vi "Begin.vi"() -> (1 "CameraDevRef":T1)   [LabVIEW 2011]
doc: "Called before other user functions, this VI is expected to open initial I/O refnums, load in file data, and do all program initialization. Notice that the <B>error out</B> terminal is simply used for data flow. Wiring it to other structures or subVIs ensures that this VI runs first."
uses:
  <vilib>/Rock Robotics/WPI/Camera/WPI_CameraDevRef.ctl
  <vilib>/Rock Robotics/SystemInterfaces/AI/FPGA_AIChannel.ctl
  <vilib>/Rock Robotics/SystemInterfaces/DIO/FPGA_DIOPWMChannel.ctl
  Robot Global Data.vi
  <vilib>/Rock Robotics/WPI/MotorControl/WPI_MotorControlOpen Jaguar.vi
  <vilib>/Rock Robotics/WPI/MotorControl/WPI_MotorControlOpen Victor.vi
  <vilib>/Rock Robotics/WPI/Joystick/WPI_JoystickDeviceEnum.ctl
  <vilib>/Rock Robotics/SystemInterfaces/DIO/FPGA_DIORelayChannel.ctl
  <vilib>/Rock Robotics/WPI/Relay/WPI_RelayDirection.ctl
  <vilib>/Rock Robotics/SystemInterfaces/Typedef/FPGA_TypedefDigitalModule.ctl
  <vilib>/Rock Robotics/WPI/Counter/WPI_CounterDigitalInputToDigitalSource.vi
  <vilib>/Rock Robotics/SystemInterfaces/DIO/FPGA_DIOChannel.ctl
  <vilib>/Rock Robotics/WPI/Encoder/WPI_EncoderType.ctl
  <vilib>/Rock Robotics/SystemInterfaces/AI/FPGA_AIGyroChannel.ctl
  <vilib>/Rock Robotics/SystemInterfaces/Typedef/FPGA_TypedefAnalogModule.ctl
  <vilib>/Utility/file.llb/Read From Spreadsheet File (DBL).vi
  <vilib>/Rock Robotics/WPI/Relay/WPI_RelayValue.ctl
panel:
  out "AutonArray":dbl[][](array[numeric])
  out "Path and file":string
  in  "Balls In Robot At Start":dbl
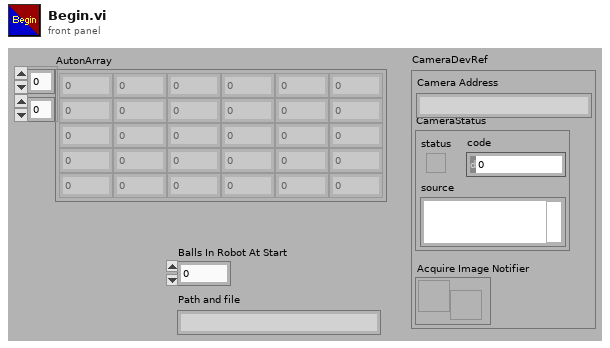
[diagram p1: front panel]
types:
  T1 = typedef "WPI_CameraDevRef.ctl" = cluster{"Camera Address":string, "CameraStatus":errorcluster, "Acquire Image Notifier":refnum<notifier>}
  T2 = typedef "FPGA_DIOPWMChannel.ctl" = enum8{"PWM 1", "PWM 2", "PWM 3", "PWM 4", "PWM 5", "PWM 6", "PWM 7", "PWM 8", "PWM 9", "PWM 10", "Invalid"}
  T3 = typedef "FPGA_AIChannel.ctl" = enum8{"AI 1", "AI 2", "AI 3", "AI 4", "AI 5", "AI 6", "AI 7", "AI 8", "Invalid"}
  T4 = typedef "WPI_CameraImageSize.ctl" = enum16{"640x480", "320x240", "160x120"}
  T5 = cluster{"fps":i32, "compression":i32, "Image Size":T4}
  T6 = typedef "WPI_CameraWhite Balance Values.ctl" = enum16{"Auto", "Fixed indoor", "Fixed outdoor 1", "Fixed outdoor 2", "Fixed fluorescent 1", "Fixed fluorescent 2", "Hold current"}
  T7 = typedef "WPI_CameraExposure Values.ctl" = enum16{"Auto", "Flicker-free 50 Hz", "Flicker-free 60 Hz", "Hold current"}
  T8 = typedef "FPGA_TypedefDigitalModule.ctl" = enum16{"Digital Module 1", "Digital Module 2"}
  T9 = typedef "WPI_ServoDeviceRef.ctl" = cluster{"DeviceStatus":errorcluster, "Digital Module":T8, "PWM Channel":T2, "DeadBand":T10}
  T10 = typedef "WPI_PWMDeadband.ctl" = cluster{"Name":string, "maxPositivePwm":i32, "minPositivePwm":i32, "centerPwm":i32, "maxNegativePwm":i32, "minNegativePwm":i32, "angularRange":u16}
  T11 = typedef "WPI_MotorControlDeviceRef.ctl" = cluster{"DeviceStatus":errorcluster, "Type":enum16{"PWM", "CAN"}, "PWM":cluster{"Digital Module":T8, "PWM Channel":T2, "DeadBand":T10}, "CAN":cluster{"Device Number":u8, "Control Mode":T12, "Semaphore":T13, "Max Vout":dbl}, "Invert":bool, "TransformRef":T14, "InvTransformRef":T14}
  T12 = typedef "WPI_CANJaguar_ControlMode.ctl" = enum8{"Percent VBus", "Current", "Speed", "Position", "Voltage"}
  T13 = typedef "Semaphore RefNum" = refnum<k1>
  T14 = typedef "WPI_PWMTransform_ConPane.ctl" = refnum<vi>
  T15 = typedef "WPI_RelayValue.ctl" = enum16{"Off", "On", "Forward", "Reverse"}
  T16 = typedef "FPGA_DIORelayChannel.ctl" = enum8{"Relay 1", "Relay 2", "Relay 3", "Relay 4", "Relay 5", "Relay 6", "Relay 7", "Relay 8", "Invalid"}
  T17 = typedef "WPI_RelayDirection.ctl" = enum16{"Both directions", "Forward only", "Reverse only"}
  T18 = typedef "WPI_JoystickDeviceEnum.ctl" = enum16{"USB 1", "USB 2", "USB 3", "USB 4", "Kinect 1", "Kinect 2"}
  T19 = typedef "WPI_JoystickDevRef.ctl" = cluster{"Device":T18}
  T20 = typedef "WPI_RelayDevRef.ctl" = cluster{"DevStatus":errorcluster, "Relay Channel":T16, "Digital Module":T8, "Relay Direction":T17}
  T21 = typedef "WPI_AnalogChannelDevRef.ctl" = cluster{"DevStatus":errorcluster, "Analog Module":T22, "Analog Channel":T3}
  T22 = typedef "FPGA_TypedefAnalogModule.ctl" = enum16{"Analog Module 1", "Analog Module 2"}
  T23 = typedef "FPGA_AIGyroChannel.ctl" = enum8{"AI 1", "AI 2", "Invalid"}
  T24 = typedef "WPI_EncoderType.ctl" = enum16{"1x", "2x", "4x"}
  T25 = typedef "FPGA_DIOChannel.ctl" = enum8{"DIO 1", "DIO 2", "DIO 3", "DIO 4", "DIO 5", "DIO 6", "DIO 7", "DIO 8", "DIO 9", "DIO 10", "DIO 11", "DIO 12", "DIO 13", "DIO 14", "Invalid"}
  T26 = typedef "WPI_DigitalInputDevRef.ctl" = cluster{"DevStatus":errorcluster, "DIO Channel":T25, "Digital Module":T8}
  T27 = typedef "FPGA_CounterEncoderSourceConvertionLVSourceType.ctl" = cluster{"DevStatus":errorcluster, "AnalogTriggerMode?":bool, "DigitalMode":cluster{"Digital Module":T8, "DIO Channel":T28}, "AnalogTriggerMode":cluster{"AnalogTriggerIndex":T29, "OutputType":T30}}
  T28 = typedef "FPGA_DIODigitalSourceChannel.ctl" = enum8{"DIO 1", "DIO 2", "DIO 3", "DIO 4", "DIO 5", "DIO 6", "DIO 7", "DIO 8", "DIO 9", "DIO 10", "DIO 11", "DIO 12", "DIO 13", "DIO 14", "Disabled"}
  T29 = typedef "FPGA_AnalogTriggerIndex.ctl" = enum8{"Trig 0", "Trig 1", "Trig 2", "Trig 3", "Trig 4", "Trig 5", "Trig 6", "Trig 7", "Invalid"}
  T30 = typedef "FPGA_AnalogTriggerOutType.ctl" = enum16{"InWindow", "TriggerState", "Rising", "Falling"}
  T31 = typedef "WPI_EncoderDevRef.ctl" = cluster{"DevStatus":errorcluster, "EncoderIndex":T32, "CounterIndex":T33, "DistancePerCount":dbl, "Decoding Type":T24}
  T32 = typedef "FPGA_EncoderIdx.ctl" = enum8{"Enc 0", "Enc 1", "Enc 2", "Enc 3", "Invalid"}
  T33 = typedef "FPGA_CounterCtrSystemIndex.ctl" = enum8{"Ctr 0", "Ctr 1", "Ctr 2", "Ctr 3", "Ctr 4", "Ctr 5", "Ctr 6", "Ctr 7", "Invalid"}
  T34 = typedef "WPI_GyroDevRef.ctl" = cluster{"DevStatus":errorcluster, "Analog Module":T22, "Analog Channel":T3, "Offset":dbl, "Gain (VoltsPerDegree/Second)":dbl}
  T35 = typedef "WPI_UltrasonicDeviceRef.ctl" = cluster{"DevStatus":errorcluster, "Ping Digital Module":T8, "Echo Digital Module":T8, "Ping Channel":T25, "Echo Channel":T25, "CntIndex":T33}
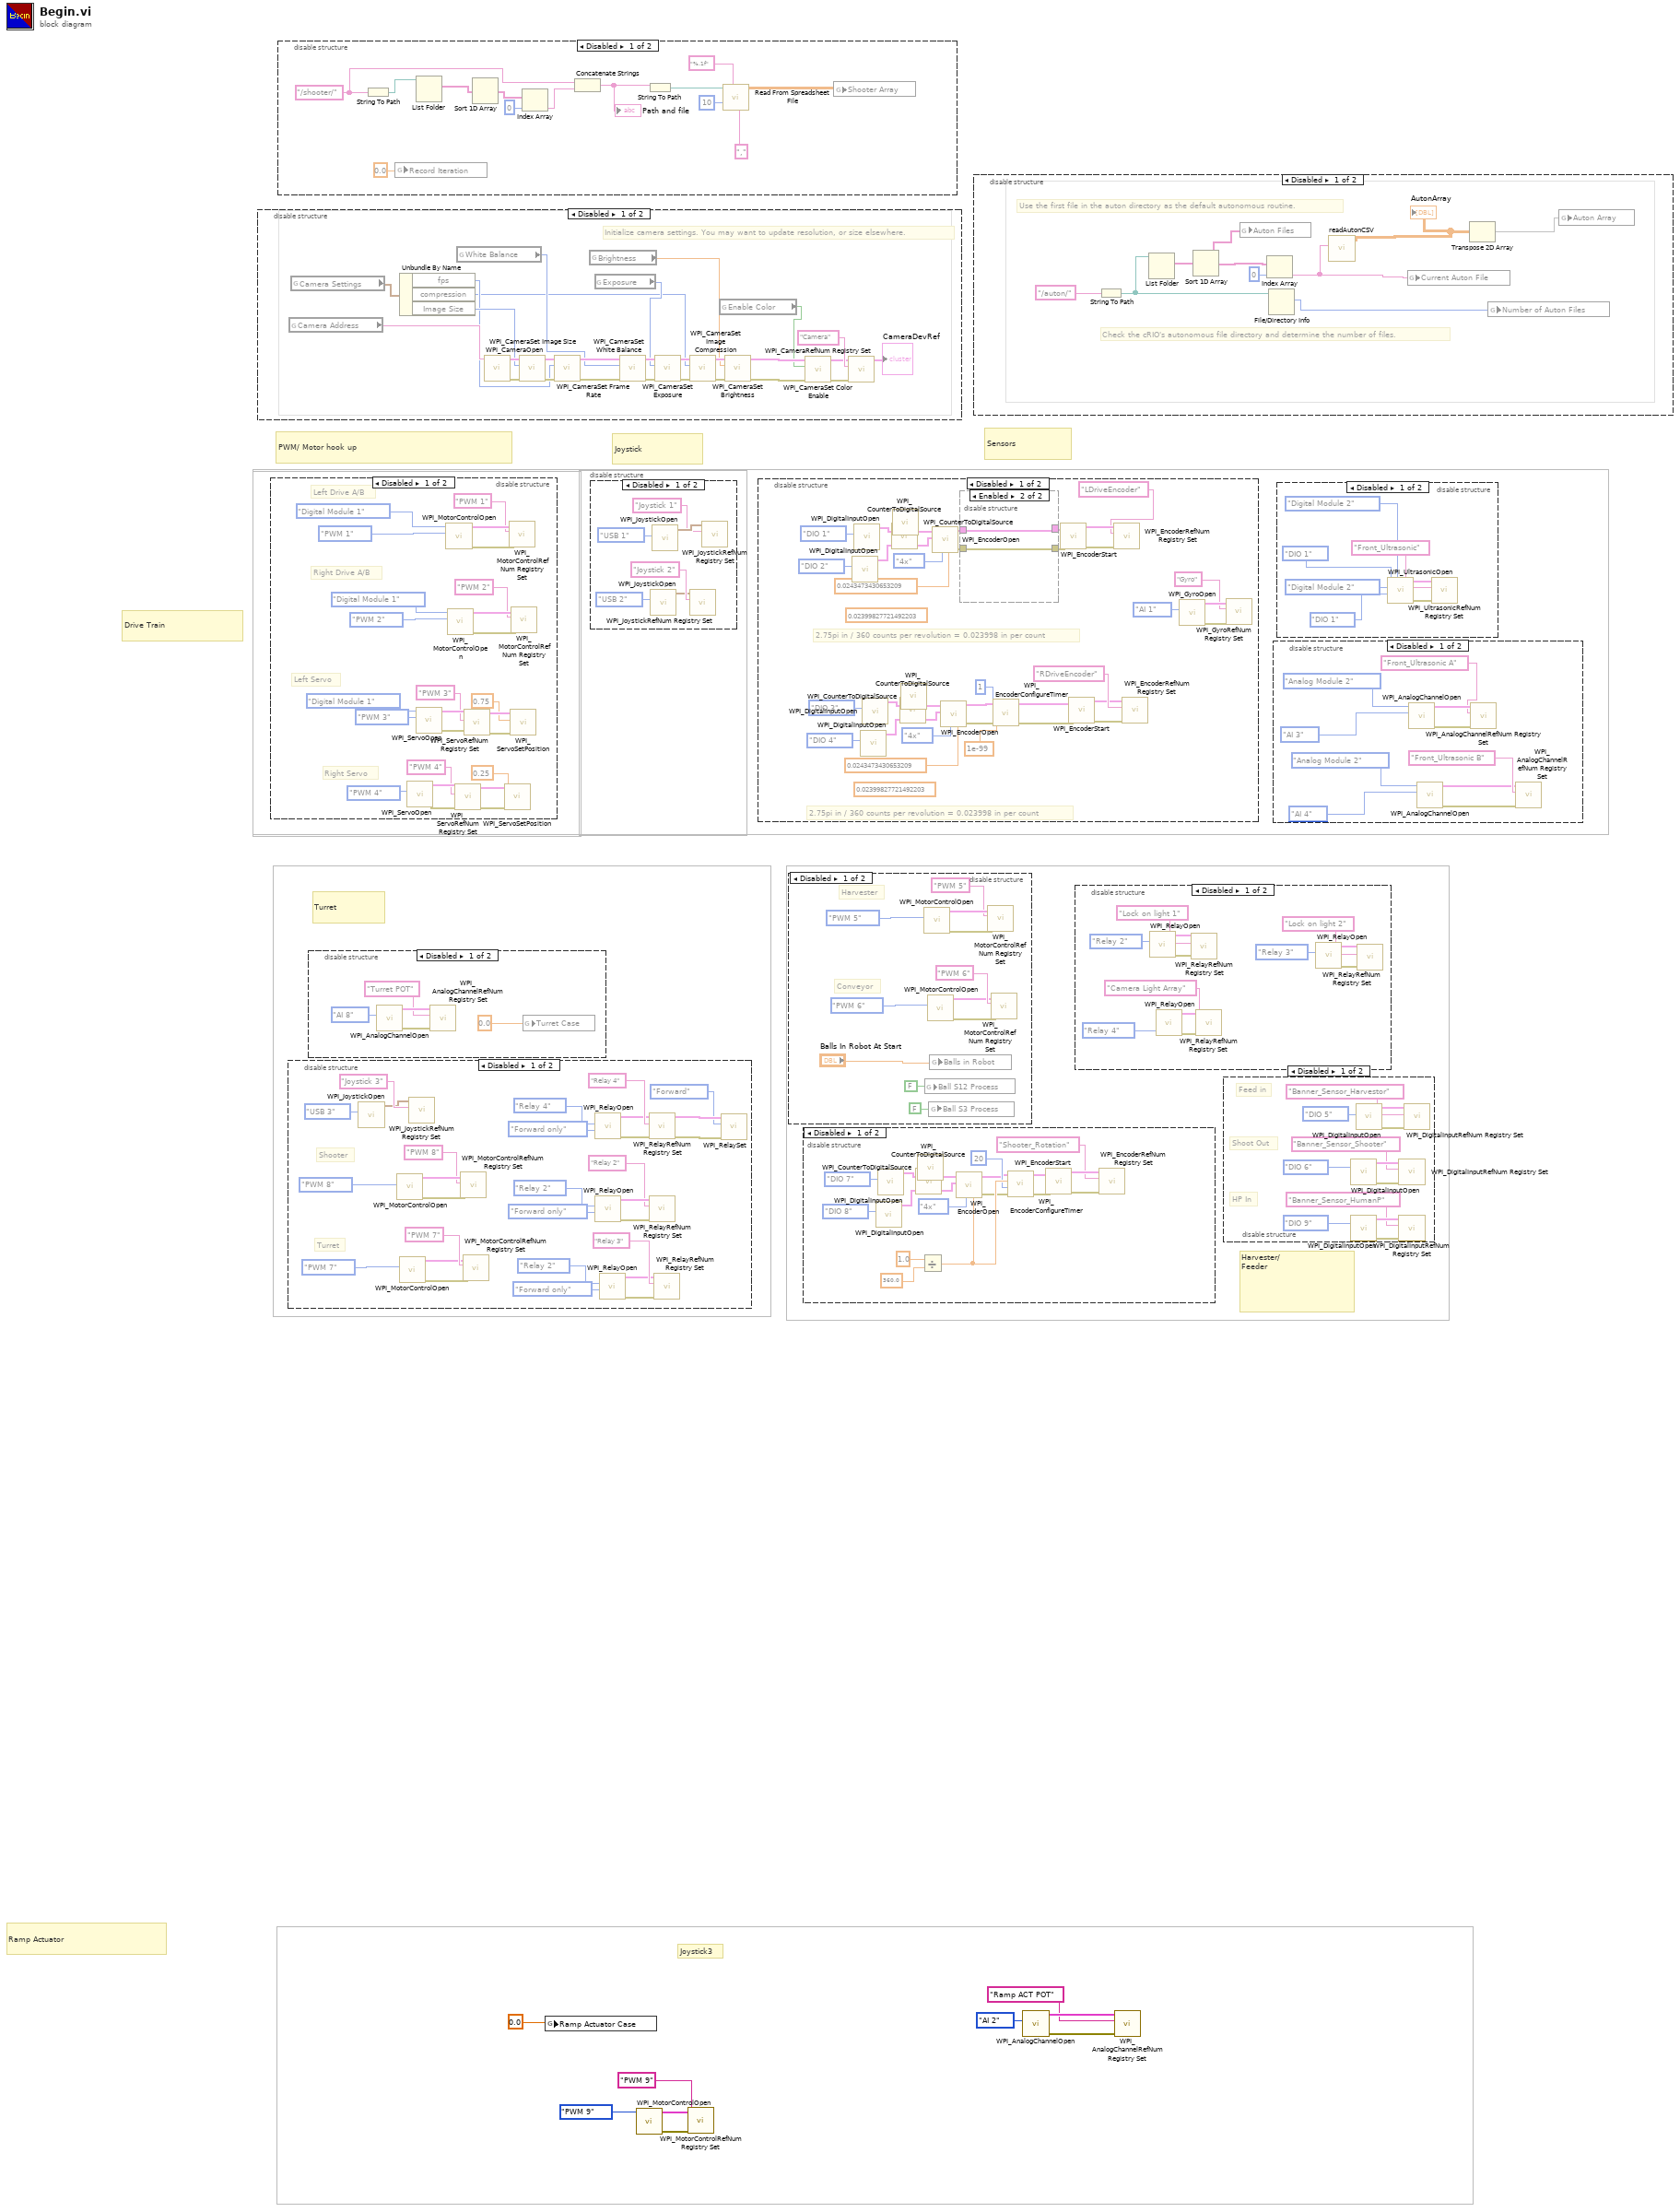
[diagram p0: block diagram]
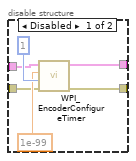
[diagram p9: hidden frame]
diagram:
  # "Harvester/\nFeeder"
  # "Joystick3"
  # "Turret"
  # "Ramp Actuator"
  # "Drive Train"
  # "Sensors"
  # "Joystick"
  # "PWM/ Motor hook up"
  n1 = disable-structure shown="Disabled" {
    frame Disabled {
      # "Initialize camera settings. You may want to update resolution, or size elsewhere."
      n2 = global read "Robot Global Data.vi" "Camera Address"() -> (w23:string)
      n3 = global read "Robot Global Data.vi" "Camera Settings"() -> (w22:T5)
      n4 = Unbundle By Name(w22) -> ("fps"=w20:i32, "compression"=w17:i32, "Image Size"=w21:T4)
      n5 = global read "Robot Global Data.vi" "White Balance"() -> (w19:T6)
      n6 = call <vilib>:"WPI_CameraOpen.vi"("Camera Address"=w23) -> ("error out"=w29:errorcluster, "CameraDevRef"=w30:T1)  [unwired: 1 in, 8 out]
      n7 = call <vilib>:"WPI_CameraSet Image Size.vi"("error in (no error)"=w29, "Image Size"=w21, "CameraDevRef"=w30) -> ("error out"=w28:errorcluster, "CameraDevRef Out"=w31:T1)  [unwired: 7 out]
      n8 = call <vilib>:"WPI_CameraSet Frame Rate.vi"("error in (no error)"=w28, "Frame Rate (fps)"=w20, "CameraDevRef"=w31) -> ("error out"=w27:errorcluster, "CameraDevRef Out"=w33:T1)  [unwired: 7 out]
      n9 = global read "Robot Global Data.vi" "Brightness"() -> (w16:dbl)
      n10 = global read "Robot Global Data.vi" "Exposure"() -> (w18:T7)
      n11 = call <vilib>:"WPI_CameraSet White Balance.vi"("error in (no error)"=w27, "White Balance"=w19, "CameraDevRef"=w33) -> ("error out"=w26:errorcluster, "CameraDevRef Out"=w32:T1)  [unwired: 7 out]
      n12 = call <vilib>:"WPI_CameraSet Exposure.vi"("error in (no error)"=w26, "Exposure"=w18, "CameraDevRef"=w32) -> ("error out"=w25:errorcluster, "CameraDevRef Out"=w35:T1)  [unwired: 7 out]
      n13 = call <vilib>:"WPI_CameraSet Image Compression.vi"("error in (no error)"=w25, "Compression"=w17, "CameraDevRef"=w35) -> ("error out"=w24:errorcluster, "CameraDevRef Out"=w34:T1)  [unwired: 7 out]
      n14 = global read "Robot Global Data.vi" "Enable Color"() -> (w11:bool)
      n15 = call <vilib>:"WPI_CameraSet Brightness.vi"("error in (no error)"=w24, "Brightness"=w16, "CameraDevRef"=w34) -> ("error out"=w14:errorcluster, "CameraDevRef Out"=w15:T1)  [unwired: 7 out]
      n16 = call <vilib>:"WPI_CameraSet Color Enable.vi"("error in (no error)"=w14, "Color Enabled"=w11, "CameraDevRef"=w15) -> ("error out"=w12:errorcluster, "CameraDevRef Out"=w13:T1)  [unwired: 7 in]
      n17 = call <vilib>:"WPI_CameraRefNum Registry Set.vi"("error in (no error)"=w12, "refnum name"="Camera", "CameraDevRef"=w13) -> ("CameraDevRef"=→"CameraDevRef":T1)  [unwired: 8 out]
    }
    frame Enabled {
    }
  }
  n18 = disable-structure shown="Disabled" {
    frame Disabled {
      # "Right Drive A/B"
      # "Left Drive A/B"
      # "Right Servo"
      # "Left Servo"
      n19 = call <vilib>:"WPI_ServoOpen.vi"("PWM Channel"=FPGA_DIOPWMChannel."PWM 4") -> ("error out"=w43:errorcluster, "ServoDeviceRef"=w58:T9)  [unwired: 9 in]
      n20 = call <vilib>:"WPI_ServoOpen.vi"("PWM Channel"=FPGA_DIOPWMChannel."PWM 3", "Digital Module (Module 1)"=FPGA_TypedefDigitalModule."Digital Module 1") -> ("error out"=w44:errorcluster, "ServoDeviceRef"=w60:T9)  [unwired: 8 in]
      n21 = call-poly <vilib>:"WPI_MotorControlOpen.vi"("PWM Channel"=FPGA_DIOPWMChannel."PWM 1", "Digital Module (Module 1)"=FPGA_TypedefDigitalModule."Digital Module 1") -> ("error out"=w48:errorcluster, "MotorControlDeviceRef"=w51:T11)  [unwired: 8 in]
      n22 = call-poly <vilib>:"WPI_MotorControlOpen.vi"("PWM Channel"=FPGA_DIOPWMChannel."PWM 2", "Digital Module (Module 1)"=FPGA_TypedefDigitalModule."Digital Module 1") -> ("error out"=w49:errorcluster, "MotorControlDeviceRef"=w54:T11)  [unwired: 8 in]
      n23 = call <vilib>:"WPI_ServoRefNum Registry Set.vi"("error in (no error)"=w43, "refnum name"="PWM 4", "ServoDeviceRef"=w58) -> ("error out"=w41:errorcluster, "ServoDeviceRef"=w42:T9)  [unwired: 7 in]
      n24 = call <vilib>:"WPI_ServoRefNum Registry Set.vi"("error in (no error)"=w44, "refnum name"="PWM 3", "ServoDeviceRef"=w60) -> ("error out"=w39:errorcluster, "ServoDeviceRef"=w40:T9)  [unwired: 7 in]
      n25 = call <vilib>:"WPI_ServoSetPosition.vi"("error in (no error)"=w41, "Position"=0.25, "ServoDeviceRef"=w42) -> ()  [unwired: 7 in, 2 out]
      n26 = call <vilib>:"WPI_MotorControlRefNum Registry Set.vi"("error in (no error)"=w48, "refnum name"="PWM 1", "MotorControlDevRef"=w51) -> ()  [unwired: 7 in, 2 out]
      n27 = call <vilib>:"WPI_ServoSetPosition.vi"("error in (no error)"=w39, "Position"=0.75, "ServoDeviceRef"=w40) -> ()  [unwired: 7 in, 2 out]
      n28 = call <vilib>:"WPI_MotorControlRefNum Registry Set.vi"("error in (no error)"=w49, "refnum name"="PWM 2", "MotorControlDevRef"=w54) -> ()  [unwired: 7 in, 2 out]
    }
    frame Enabled {
    }
  }
  n29 = disable-structure shown="Disabled" {
    frame Disabled {
      w65 = "/shooter/" ("string")
      n30 = String To Path(string=w65) -> (path=w74:path)
      n31 = global write "Robot Global Data.vi" "Record Iteration"(0.0 ("Record Iteration")) -> ()
      n32 = List Folder(path=w74) -> (filenames=w73:string[])  [unwired: 1 in, 5 out]
      n33 = Sort 1D Array(array=w73) -> (sorted array=w72:string[])
      n34 = Index Array(array=w72, index=0) -> (element=w64:string)
      n35 = Concatenate Strings(w65, w64) -> (w67:string)
      "Path and file" <- w67
      n36 = String To Path(string=w67) -> (path=w66:path)
      n37 = call-poly <vilib>:"Read From Spreadsheet File.vi"("delimiter (\\t)"="," ("delimiter (\\t)"), "format (%.3f)"="%.1f", "number of rows (all:-1)"=10, "file path (dialog if empty)"=w66) -> ("all rows"=w63:dbl[][])  [unwired: 1 in, 6 out]
      n38 = global write "Robot Global Data.vi" "Shooter Array"(w63) -> ()
    }
    frame Enabled {
    }
  }
  n39 = disable-structure shown="Disabled" {
    frame Disabled {
      # "Turret"
      # "Shooter"
      n40 = call <vilib>:"WPI_JoystickOpen.vi"("JoystickDevice"=WPI_JoystickDeviceEnum."USB 3") -> ("JoystickDevRef"=w102:T19)  [unwired: 10 in]
      n41 = call-poly <vilib>:"WPI_MotorControlOpen.vi"("PWM Channel"=FPGA_DIOPWMChannel."PWM 8") -> ("error out"=w79:errorcluster, "MotorControlDeviceRef"=w81:T11)  [unwired: 9 in]
      n42 = call-poly <vilib>:"WPI_MotorControlOpen.vi"("PWM Channel"=FPGA_DIOPWMChannel."PWM 7") -> ("error out"=w78:errorcluster, "MotorControlDeviceRef"=w76:T11)  [unwired: 9 in]
      n43 = call <vilib>:"WPI_JoystickRefNum Registry Set.vi"("refnum name"="Joystick 3", "JoystickDevRef"=w102) -> ()  [unwired: 8 in, 2 out]
      n44 = call <vilib>:"WPI_MotorControlRefNum Registry Set.vi"("error in (no error)"=w79, "refnum name"="PWM 8", "MotorControlDevRef"=w81) -> ()  [unwired: 7 in, 2 out]
      n45 = call <vilib>:"WPI_MotorControlRefNum Registry Set.vi"("error in (no error)"=w78, "refnum name"="PWM 7", "MotorControlDevRef"=w76) -> ()  [unwired: 7 in, 2 out]
      n46 = call <vilib>:"WPI_RelayOpen.vi"("Relay Direction"=WPI_RelayDirection."Forward only", "Relay Channel"=FPGA_DIORelayChannel."Relay 4") -> ("error out"=w87:errorcluster, "RelayDevRef"=w86:T20)  [unwired: 8 in]
      n47 = call <vilib>:"WPI_RelayOpen.vi"("Relay Direction"=WPI_RelayDirection."Forward only", "Relay Channel"=FPGA_DIORelayChannel."Relay 2") -> ("error out"=w99:errorcluster, "RelayDevRef"=w100:T20)  [unwired: 8 in]
      n48 = call <vilib>:"WPI_RelayOpen.vi"("Relay Direction"=WPI_RelayDirection."Forward only", "Relay Channel"=FPGA_DIORelayChannel."Relay 2") -> ("error out"=w92:errorcluster, "RelayDevRef"=w91:T20)  [unwired: 8 in]
      n49 = call <vilib>:"WPI_RelayRefNum Registry Set.vi"("error in (no error)"=w87, "refnum name"="Relay 4", "RelayDevRef"=w86) -> ("error out"=w84:errorcluster, "RelayDevRef"=w85:T20)  [unwired: 7 in]
      n50 = call <vilib>:"WPI_RelayRefNum Registry Set.vi"("error in (no error)"=w99, "refnum name"="Relay 2", "RelayDevRef"=w100) -> ()  [unwired: 7 in, 2 out]
      n51 = call <vilib>:"WPI_RelayRefNum Registry Set.vi"("error in (no error)"=w92, "refnum name"="Relay 3", "RelayDevRef"=w91) -> ()  [unwired: 7 in, 2 out]
      n52 = call <vilib>:"WPI_RelaySet.vi"("error in (no error)"=w84, "RelayValue"=WPI_RelayValue."Forward", "RelayDevRef"=w85) -> ()  [unwired: 7 in, 2 out]
    }
    frame Enabled {
    }
  }
  n53 = disable-structure shown="Disabled" {
    frame Disabled {
      n54 = call <vilib>:"WPI_AnalogChannelOpen.vi"("Analog Channel"=FPGA_AIChannel."AI 8") -> ("error out"=w107:errorcluster, "AIDeviceRef"=w108:T21)  [unwired: 9 in]
      n55 = call <vilib>:"WPI_AnalogChannelRefNum Registry Set.vi"("error in (no error)"=w107, "refnum name"="Turret POT", "AIDeviceRef"=w108) -> ()  [unwired: 7 in, 2 out]
      n56 = global write "Robot Global Data.vi" "Turret Case"(0.0 ("Return To Home Case")) -> ()
    }
    frame Enabled {
    }
  }
  n57 = global write "Robot Global Data.vi" "Ramp Actuator Case"(0.0 ("Ramp Actuator Case")) -> ()
  n58 = disable-structure shown="Disabled" {
    frame Disabled {
      n59 = call <vilib>:"WPI_JoystickOpen.vi"("JoystickDevice"=WPI_JoystickDeviceEnum."USB 2") -> ("JoystickDevRef"=w111:T19)  [unwired: 10 in]
      n60 = call <vilib>:"WPI_JoystickOpen.vi"("JoystickDevice"=WPI_JoystickDeviceEnum."USB 1") -> ("JoystickDevRef"=w114:T19)  [unwired: 10 in]
      n61 = call <vilib>:"WPI_JoystickRefNum Registry Set.vi"("refnum name"="Joystick 2", "JoystickDevRef"=w111) -> ()  [unwired: 8 in, 2 out]
      n62 = call <vilib>:"WPI_JoystickRefNum Registry Set.vi"("refnum name"="Joystick 1", "JoystickDevRef"=w114) -> ()  [unwired: 8 in, 2 out]
    }
    frame Enabled {
    }
  }
  n63 = call-poly <vilib>:"WPI_MotorControlOpen.vi"("PWM Channel"=FPGA_DIOPWMChannel."PWM 9") -> ("error out"=w3:errorcluster, "MotorControlDeviceRef"=w4:T11)  [unwired: 9 in]
  n64 = call <vilib>:"WPI_MotorControlRefNum Registry Set.vi"("error in (no error)"=w3, "refnum name"="PWM 9", "MotorControlDevRef"=w4) -> ()  [unwired: 7 in, 2 out]
  n65 = disable-structure shown="Disabled" {
    frame Disabled {
      (unwired) 0.02399827721492203 ("DistancePerCount")
      (unwired) 0.02399827721492203 ("DistancePerCount")
      # "2.75pi in / 360 counts per revolution = 0.023998 in per count"
      # "2.75pi in / 360 counts per revolution = 0.023998 in per count"
      n66 = call <vilib>:"WPI_DigitalInputOpen.vi"("DIO Channel"=FPGA_DIOChannel."DIO 2") -> ("DigitalInputDevRef"=w142:T26)  [unwired: 9 in, 1 out]
      n67 = call <vilib>:"WPI_DigitalInputOpen.vi"("DIO Channel"=FPGA_DIOChannel."DIO 1") -> ("DigitalInputDevRef"=w139:T26)  [unwired: 9 in, 1 out]
      n68 = call <vilib>:"WPI_DigitalInputOpen.vi"("DIO Channel"=FPGA_DIOChannel."DIO 4") -> ("DigitalInputDevRef"=w133:T26)  [unwired: 9 in, 1 out]
      n69 = call <vilib>:"WPI_DigitalInputOpen.vi"("DIO Channel"=FPGA_DIOChannel."DIO 3") -> ("DigitalInputDevRef"=w136:T26)  [unwired: 9 in, 1 out]
      n70 = call-poly <vilib>:"WPI_CounterToDigitalSource.vi"("DigitalInputDevRef"=w142) -> ("Digital Source"=w143:T27)  [unwired: 6 in]
      n71 = call-poly <vilib>:"WPI_CounterToDigitalSource.vi"("DigitalInputDevRef"=w139) -> ("Digital Source"=w138:T27)  [unwired: 6 in]
      n72 = call-poly <vilib>:"WPI_CounterToDigitalSource.vi"("DigitalInputDevRef"=w133) -> ("Digital Source"=w132:T27)  [unwired: 6 in]
      n73 = call-poly <vilib>:"WPI_CounterToDigitalSource.vi"("DigitalInputDevRef"=w136) -> ("Digital Source"=w137:T27)  [unwired: 6 in]
      n74 = call <vilib>:"WPI_EncoderOpen.vi"("DistancePerCount"=0.0243473430653209, "Decoding Type"=WPI_EncoderType."4x", "BSource"=w143, "ASource"=w138) -> ("error out"=w145:errorcluster, "EncoderDevRef"=w146:T31)  [unwired: 6 in]
      n75 = call <vilib>:"WPI_EncoderOpen.vi"("DistancePerCount"=0.0243473430653209, "Decoding Type"=WPI_EncoderType."4x", "BSource"=w132, "ASource"=w137) -> ("error out"=w129:errorcluster, "EncoderDevRef"=w128:T31)  [unwired: 6 in]
      n76 = disable-structure shown="Enabled" {
        disable-tunnel: [w156 w157] -> w148
        disable-tunnel: [w155 w158] -> w147
        disable-tunnel: w146 -> [w152 w158]
        disable-tunnel: w145 -> [w151 w157]
        frame Disabled {
          n77 = call <vilib>:"WPI_EncoderConfigureTimer.vi"("error in (no error)"=w151, "Number Samples to Average"=u8 1, "Minimum Rate"=1e-99, "EncoderDevRef"=w152) -> ("error out"=w156:errorcluster, "EncoderDevRef"=w155:T31)  [unwired: 6 in]
        }
        frame Enabled {
        }
      }
      n78 = call <vilib>:"WPI_EncoderConfigureTimer.vi"("error in (no error)"=w129, "Number Samples to Average"=u8 1, "Minimum Rate"=1e-99, "EncoderDevRef"=w128) -> ("error out"=w124:errorcluster, "EncoderDevRef"=w125:T31)  [unwired: 6 in]
      n79 = call <vilib>:"WPI_EncoderStart.vi"("error in (no error)"=w148, "EncoderDevRef"=w147) -> ("error out"=w150:errorcluster, "EncoderDevRef"=w149:T31)  [unwired: 8 in]
      n80 = call <vilib>:"WPI_EncoderStart.vi"("error in (no error)"=w124, "EncoderDevRef"=w125) -> ("error out"=w122:errorcluster, "EncoderDevRef"=w123:T31)  [unwired: 8 in]
      n81 = call <vilib>:"WPI_EncoderRefNum Registry Set.vi"("error in (no error)"=w150, "refnum name"="LDriveEncoder", "EncoderDevRef"=w149) -> ()  [unwired: 7 in, 2 out]
      n82 = call <vilib>:"WPI_EncoderRefNum Registry Set.vi"("error in (no error)"=w122, "refnum name"="RDriveEncoder", "EncoderDevRef"=w123) -> ()  [unwired: 7 in, 2 out]
      n83 = call <vilib>:"WPI_GyroOpen.vi"("Analog Channel"=FPGA_AIGyroChannel."AI 1") -> ("error out"=w118:errorcluster, "GyroDevRef"=w117:T34)  [unwired: 8 in, 1 out]
      n84 = call <vilib>:"WPI_GyroRefNum Registry Set.vi"("error in (no error)"=w118, "refnum name"="Gyro", "GyroDevRef"=w117) -> ()  [unwired: 7 in, 2 out]
    }
    frame Enabled {
    }
  }
  n85 = disable-structure shown="Disabled" {
    frame Disabled {
      # "Harvester"
      # "Conveyor"
      n86 = call-poly <vilib>:"WPI_MotorControlOpen.vi"("PWM Channel"=FPGA_DIOPWMChannel."PWM 5") -> ("error out"=w166:errorcluster, "MotorControlDeviceRef"=w168:T11)  [unwired: 9 in]
      n87 = global write "Robot Global Data.vi" "Ball S12 Process"(FALSE ("Ball S12 Process")) -> ()
      n88 = call-poly <vilib>:"WPI_MotorControlOpen.vi"("PWM Channel"=FPGA_DIOPWMChannel."PWM 6") -> ("error out"=w165:errorcluster, "MotorControlDeviceRef"=w163:T11)  [unwired: 9 in]
      n89 = global write "Robot Global Data.vi" "Ball S3 Process"(FALSE ("Ball S3 Process")) -> ()
      n90 = global write "Robot Global Data.vi" "Balls in Robot"("Balls In Robot At Start") -> ()
      n91 = call <vilib>:"WPI_MotorControlRefNum Registry Set.vi"("error in (no error)"=w166, "refnum name"="PWM 5", "MotorControlDevRef"=w168) -> ()  [unwired: 7 in, 2 out]
      n92 = call <vilib>:"WPI_MotorControlRefNum Registry Set.vi"("error in (no error)"=w165, "refnum name"="PWM 6", "MotorControlDevRef"=w163) -> ()  [unwired: 7 in, 2 out]
    }
    frame Enabled {
    }
  }
  n93 = disable-structure shown="Disabled" {
    frame Disabled {
      n94 = call <vilib>:"WPI_DigitalInputOpen.vi"("DIO Channel"=FPGA_DIOChannel."DIO 8") -> ("DigitalInputDevRef"=w174:T26)  [unwired: 9 in, 1 out]
      n95 = call <vilib>:"WPI_DigitalInputOpen.vi"("DIO Channel"=FPGA_DIOChannel."DIO 7") -> ("DigitalInputDevRef"=w171:T26)  [unwired: 9 in, 1 out]
      n96 = call-poly <vilib>:"WPI_CounterToDigitalSource.vi"("DigitalInputDevRef"=w174) -> ("Digital Source"=w175:T27)  [unwired: 6 in]
      n97 = call-poly <vilib>:"WPI_CounterToDigitalSource.vi"("DigitalInputDevRef"=w171) -> ("Digital Source"=w170:T27)  [unwired: 6 in]
      n98 = Divide(x=1.0, y=360.0) -> (x/y=w187:dbl)
      n99 = call <vilib>:"WPI_EncoderOpen.vi"("DistancePerCount"=w187, "Decoding Type"=WPI_EncoderType."4x", "BSource"=w175, "ASource"=w170) -> ("error out"=w178:errorcluster, "EncoderDevRef"=w179:T31)  [unwired: 6 in]
      n100 = call <vilib>:"WPI_EncoderConfigureTimer.vi"("error in (no error)"=w178, "Number Samples to Average"=u8 20, "Minimum Rate"=w187, "EncoderDevRef"=w179) -> ("error out"=w182:errorcluster, "EncoderDevRef"=w181:T31)  [unwired: 6 in]
      n101 = call <vilib>:"WPI_EncoderStart.vi"("error in (no error)"=w182, "EncoderDevRef"=w181) -> ("error out"=w184:errorcluster, "EncoderDevRef"=w183:T31)  [unwired: 8 in]
      n102 = call <vilib>:"WPI_EncoderRefNum Registry Set.vi"("error in (no error)"=w184, "refnum name"="Shooter_Rotation", "EncoderDevRef"=w183) -> ()  [unwired: 7 in, 2 out]
    }
    frame Enabled {
    }
  }
  n103 = disable-structure shown="Disabled" {
    frame Disabled {
      # "Check the cRIO's autonomous file directory and determine the number of files."
      # "Use the first file in the auton directory as the default autonomous routine."
      n104 = String To Path(string="/auton/") -> (path=w195:path)
      n105 = List Folder(path=w195) -> (filenames=w194:string[])  [unwired: 1 in, 5 out]
      n106 = Sort 1D Array(array=w194) -> (sorted array=w190:string[])
      n107 = global write "Robot Global Data.vi" "Auton Files"(w190) -> ()
      n108 = Index Array(array=w190, index=0) -> (element=w191:string)
      n109 = File/Directory Info(path=w195) -> (size=w192:i64)  [unwired: 1 in, 6 out]
      n110 = call "readAutonCSV.vi"("AutonFile"=w191) -> ("AutonArray"=w189:dbl[][])  [unwired: 7 in]
      "AutonArray" <- w189
      n111 = global write "Robot Global Data.vi" "Current Auton File"(w191) -> ()
      n112 = Transpose 2D Array(2D array=w189) -> (transposed array=w188:dbl[][])
      n113 = global write "Robot Global Data.vi" "Number of Auton Files"(w192) -> ()
      n114 = global write "Robot Global Data.vi" "Auton Array"(w188) -> ()
    }
    frame Enabled {
    }
  }
  n115 = call <vilib>:"WPI_AnalogChannelOpen.vi"("Analog Channel"=FPGA_AIChannel."AI 2") -> ("error out"=w8:errorcluster, "AIDeviceRef"=w9:T21)  [unwired: 9 in]
  n116 = disable-structure shown="Disabled" {
    frame Disabled {
      n117 = call <vilib>:"WPI_RelayOpen.vi"("Relay Channel"=FPGA_DIORelayChannel."Relay 2") -> ("error out"=w206:errorcluster, "RelayDevRef"=w205:T20)  [unwired: 9 in]
      n118 = call <vilib>:"WPI_RelayOpen.vi"("Relay Channel"=FPGA_DIORelayChannel."Relay 4") -> ("error out"=w208:errorcluster, "RelayDevRef"=w207:T20)  [unwired: 9 in]
      n119 = call <vilib>:"WPI_RelayRefNum Registry Set.vi"("error in (no error)"=w206, "refnum name"="Lock on light 1", "RelayDevRef"=w205) -> ()  [unwired: 7 in, 2 out]
      n120 = call <vilib>:"WPI_RelayRefNum Registry Set.vi"("error in (no error)"=w208, "refnum name"="Camera Light Array", "RelayDevRef"=w207) -> ()  [unwired: 7 in, 2 out]
      n121 = call <vilib>:"WPI_RelayOpen.vi"("Relay Channel"=FPGA_DIORelayChannel."Relay 3") -> ("error out"=w197:errorcluster, "RelayDevRef"=w198:T20)  [unwired: 9 in]
      n122 = call <vilib>:"WPI_RelayRefNum Registry Set.vi"("error in (no error)"=w197, "refnum name"="Lock on light 2", "RelayDevRef"=w198) -> ()  [unwired: 7 in, 2 out]
    }
    frame Enabled {
    }
  }
  n123 = call <vilib>:"WPI_AnalogChannelRefNum Registry Set.vi"("error in (no error)"=w8, "refnum name"="Ramp ACT POT", "AIDeviceRef"=w9) -> ()  [unwired: 7 in, 2 out]
  n124 = disable-structure shown="Disabled" {
    frame Disabled {
      # "HP In"
      # "Shoot Out"
      # "Feed in"
      n125 = call <vilib>:"WPI_DigitalInputOpen.vi"("DIO Channel"=FPGA_DIOChannel."DIO 6") -> ("error out"=w215:errorcluster, "DigitalInputDevRef"=w214:T26)  [unwired: 9 in]
      n126 = call <vilib>:"WPI_DigitalInputOpen.vi"("DIO Channel"=FPGA_DIOChannel."DIO 9") -> ("error out"=w211:errorcluster, "DigitalInputDevRef"=w210:T26)  [unwired: 9 in]
      n127 = call <vilib>:"WPI_DigitalInputOpen.vi"("DIO Channel"=FPGA_DIOChannel."DIO 5") -> ("error out"=w218:errorcluster, "DigitalInputDevRef"=w217:T26)  [unwired: 9 in]
      n128 = call <vilib>:"WPI_DigitalInputRefNum Registry Set.vi"("error in (no error)"=w215, "refnum name"="Banner_Sensor_Shooter", "DigitalInputDevRef"=w214) -> ()  [unwired: 7 in, 2 out]
      n129 = call <vilib>:"WPI_DigitalInputRefNum Registry Set.vi"("error in (no error)"=w211, "refnum name"="Banner_Sensor_HumanP", "DigitalInputDevRef"=w210) -> ()  [unwired: 7 in, 2 out]
      n130 = call <vilib>:"WPI_DigitalInputRefNum Registry Set.vi"("error in (no error)"=w218, "refnum name"="Banner_Sensor_Harvestor", "DigitalInputDevRef"=w217) -> ()  [unwired: 7 in, 2 out]
    }
    frame Enabled {
    }
  }
  n131 = disable-structure shown="Disabled" {
    frame Disabled {
      n132 = call <vilib>:"WPI_AnalogChannelOpen.vi"("Analog Channel"=FPGA_AIChannel."AI 3", "Analog Module (Module 1)"=FPGA_TypedefAnalogModule."Analog Module 2") -> ("error out"=w226:errorcluster, "AIDeviceRef"=w225:T21)  [unwired: 8 in]
      n133 = call <vilib>:"WPI_AnalogChannelOpen.vi"("Analog Channel"=FPGA_AIChannel."AI 4", "Analog Module (Module 1)"=FPGA_TypedefAnalogModule."Analog Module 2") -> ("error out"=w221:errorcluster, "AIDeviceRef"=w222:T21)  [unwired: 8 in]
      n134 = call <vilib>:"WPI_AnalogChannelRefNum Registry Set.vi"("error in (no error)"=w226, "refnum name"="Front_Ultrasonic A", "AIDeviceRef"=w225) -> ()  [unwired: 7 in, 2 out]
      n135 = call <vilib>:"WPI_AnalogChannelRefNum Registry Set.vi"("error in (no error)"=w221, "refnum name"="Front_Ultrasonic B", "AIDeviceRef"=w222) -> ()  [unwired: 7 in, 2 out]
    }
    frame Enabled {
    }
  }
  n136 = disable-structure shown="Disabled" {
    frame Disabled {
      n137 = call <vilib>:"WPI_UltrasonicOpen.vi"("Ping Digital Module (Module 1)"=FPGA_TypedefDigitalModule."Digital Module 2", "Echo DIO Channel"=FPGA_DIOChannel."DIO 1", "Echo Digital Module (Module 1)"=FPGA_TypedefDigitalModule."Digital Module 2", "Ping DIO Channel"=FPGA_DIOChannel."DIO 1") -> ("error out"=w237:errorcluster, "UltrasonicDevRef"=w236:T35)  [unwired: 6 in]
      n138 = call <vilib>:"WPI_UltrasonicRefNum Registry Set.vi"("error in (no error)"=w237, "refnum name"="Front_Ultrasonic", "UltrasonicDevRef"=w236) -> ()  [unwired: 7 in, 2 out]
    }
    frame Enabled {
    }
  }
